vi "common_generate_GLOBAL_STOP.vi"(8 "error in (no error)":errorcluster) -> (0 "error out":errorcluster)   [LabVIEW 2019]
doc: "Publishes topic \"GLOBAL STOP\" with value of True."
uses:
  common data types/common_event_data.ctl
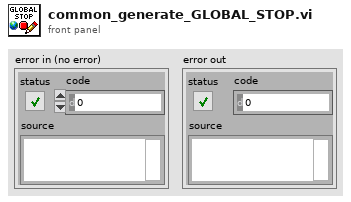
[diagram p1: front panel]
types:
  T1 = typedef "common_event_data.ctl" = cluster{"sender":string, "target":string, "msg":string, "data":variant}
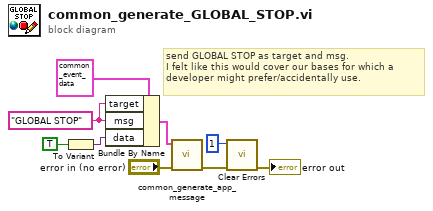
[diagram p0: block diagram]
diagram:
  w4 = "GLOBAL STOP" ("target")
  # "send GLOBAL STOP as target and msg.\nI felt like this would cover our bases for which a developer might prefer/accidentally use."
  n1 = To Variant(anything=TRUE) -> (Variant=w7:variant)
  n2 = Bundle By Name(cluster=T1 {"sender"="", "target"="GLOBAL STOP", "msg"="", "data"=variant} ("event data"), "target"=w4, "msg"=w4, "data"=w7) -> (w6:T1)
  n3 = call "common_generate_app_message.vi"("error in (no error)"="error in (no error)", "event data"=w6) -> ("error out"=w2:errorcluster)  [unwired: 9 in]
  n4 = call <vilib>:"Clear Errors.vi"("error in (no error)"=w2, "specific error code to clear (0: all)"=1) -> ("error out"=→"error out":errorcluster)  [unwired: 4 in, 1 out]
